vi "HSL to Color.vi"(8 "L (%)":dbl, 9 "S (%)":dbl, 10 "H (degrees)":dbl) -> (0 "B":u8, 1 "G":u8, 2 "R":u8, 3 "Color out":u32(colorbox)=16767232)   [LabVIEW 2021, in "Material SubVIs.lvlib"]
doc: "take HSL and convert to a color box and the RGB outputs\n\n<b>Code Developed By:</b> +\nDaniel Coons +\nTechnology Service Corporation +\nwww.tsc.com/atcs"
uses:
  Material SubVIs.lvlib
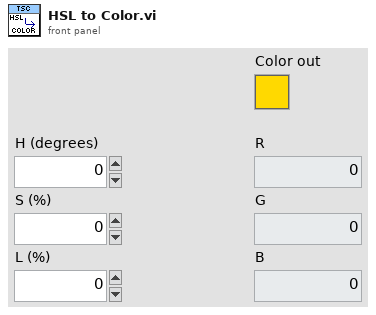
[diagram p1: front panel]
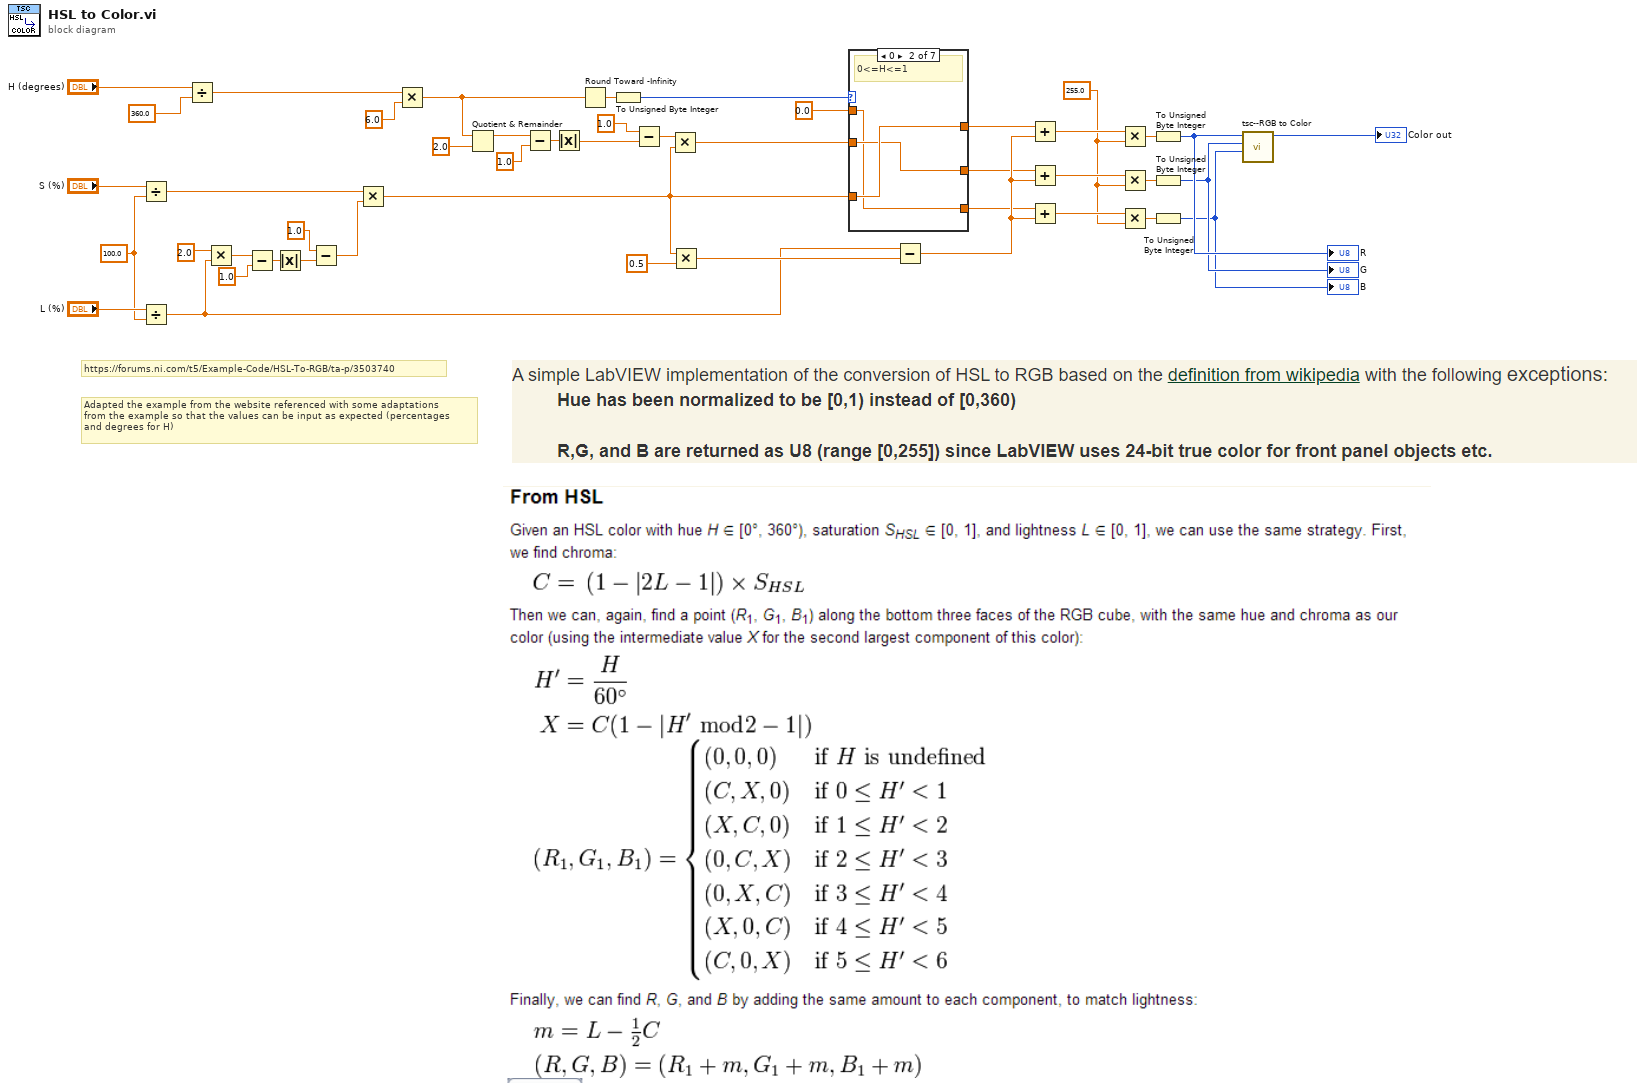
[diagram p0: block diagram]
diagram:
  w7 = 100.0 ("y")
  w5 = 255.0 ("y")
  # "Adapted the example from the website referenced with some adaptations\nfrom the example so that the values can be input as expected (percentages\nand degrees for H)"
  # "https://forums.ni.com/t5/Example-Code/HSL-To-RGB/ta-p/3503740"
  n1 = Divide(x="S (%)", y=w7) -> (x/y=w9:dbl)
  n2 = Divide(x="L (%)", y=w7) -> (x/y=w6:dbl)
  n3 = Divide(x="H (degrees)", y=360.0) -> (x/y=w11:dbl)
  n4 = Multiply(x=2.0 ("y"), y=w6) -> (x*y=w46:dbl)
  n5 = Subtract(x=w46, y=1.0) -> (x-y=w44:dbl)
  n6 = Absolute Value(x=w44) -> (abs(x)=w43:dbl)
  n7 = Subtract(x=1.0, y=w43) -> (x-y=w25:dbl)
  n8 = Multiply(x=w9, y=w25) -> (x*y=w17:dbl)
  n9 = Multiply(x=w11, y=6.0) -> (x*y=w33:dbl)
  n10 = Quotient & Remainder(x=w33, y=2.0) -> (x-y*floor(x/y)=w31:dbl)  [unwired: 1 out]
  n11 = Subtract(x=w31, y=1.0) -> (x-y=w29:dbl)
  n12 = Absolute Value(x=w29) -> (abs(x)=w28:dbl)
  n13 = Round Toward -Infinity(1:w33) -> (0:w40:dbl)
  n14 = To Unsigned Byte Integer(number=w40) -> (unsigned 8bit integer=w20:u8)
  n15 = Subtract(x=1.0, y=w28) -> (x-y=w26:dbl)
  n16 = Multiply(x=w26, y=w17) -> (x*y=w18:dbl)
  n17 = Multiply(x=w17, y=0.5) -> (x*y=w23:dbl)
  n18 = case shown="0" w20 {
    tunnel: w17 -> [_ w50 w52 w55 w57 w60 w65]
    tunnel: w18 -> [_ w49 w53 w54 w58 w62 w63]
    tunnel: 0.0 -> [w47 w48 w51 w56 w59 w61 w64]
    tunnel: [w47 w50 w53 w56 w59 w62 w65] -> w14
    tunnel: [w47 w49 w52 w55 w58 w61 w64] -> w15
    tunnel: [w47 w48 w51 w54 w57 w60 w63] -> w16
    frame Default {
      # "H undefined"
    }
    frame 0 {
      # "0<=H<=1"
    }
    frame 1 {
      # "1<=H<=2"
    }
    frame 2 {
      # "2<=H<=3"
    }
    frame 3 {
      # "3<=H<=4"
    }
    frame 4 {
      # "4<=H<=5"
    }
    frame 5 {
      # "5<=H<=6"
    }
  }
  n19 = Subtract(x=w6, y=w23) -> (x-y=w22:dbl)
  n20 = Add(x=w14, y=w22) -> (x+y=w34:dbl)
  n21 = Add(x=w15, y=w22) -> (x+y=w35:dbl)
  n22 = Add(x=w16, y=w22) -> (x+y=w36:dbl)
  n23 = Multiply(x=w34, y=w5) -> (x*y=w39:dbl)
  n24 = Multiply(x=w35, y=w5) -> (x*y=w38:dbl)
  n25 = Multiply(x=w36, y=w5) -> (x*y=w37:dbl)
  n26 = To Unsigned Byte Integer(number=w39) -> (unsigned 8bit integer=w3:u8)
  "R" <- w3
  n27 = To Unsigned Byte Integer(number=w38) -> (unsigned 8bit integer=w2:u8)
  "G" <- w2
  n28 = To Unsigned Byte Integer(number=w37) -> (unsigned 8bit integer=w1:u8)
  "B" <- w1
  n29 = call "tsc--RGB to Color.vi"("B"=w1, "G"=w2, "R"=w3) -> ("Color"=→"Color out":u32)  [unwired: 8 in]
